vi "Find Tests from Path.vi"(8 "error in (no error)":errorcluster, 10 "Project or Class Path":path, 11 "Test Case Finder In":refnum<class "Indexing Test Finder.lvclass">) -> (0 "error out":errorcluster, 3 "Test Case Finder Out":refnum<class "Indexing Test Finder.lvclass">)   [LabVIEW 2020, in "Indexing Test Finder.lvclass"]
uses:
  Indexing Test Finder.lvclass
  Test Finder/Test Finder.lvclass
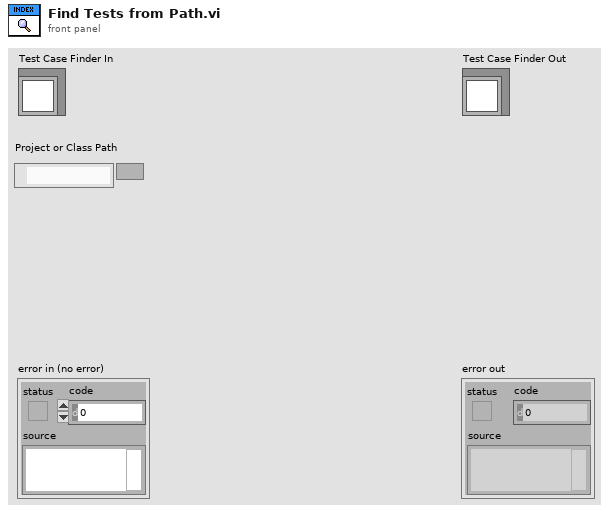
[diagram p1: front panel]
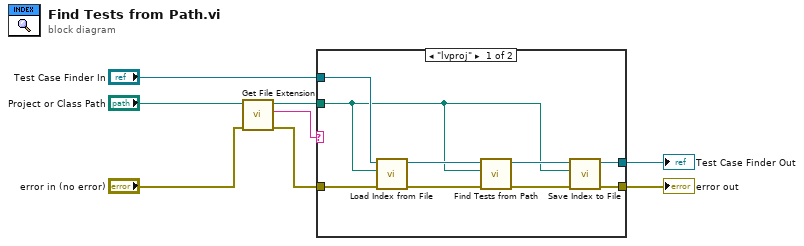
[diagram p0: block diagram]
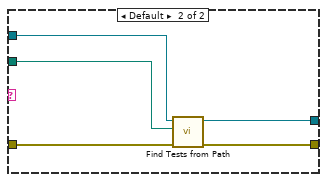
[diagram p2: hidden frame]
diagram:
  n1 = call <vilib>:"Get File Extension.vi"("error in (no error)"="error in (no error)", "file"="Project or Class Path") -> ("error out"=w4:errorcluster, "lowercase file extension"=w1:string, "dup file"=w2:path)  [unwired: 5 in, 2 out]
  n2 = case shown="\"lvproj\"" w1 {
    tunnel: "Test Case Finder In" -> [w17 w22]
    tunnel: [w13 w21] -> w6
    tunnel: [w11 w20] -> w5
    tunnel: w4 -> [w10 w19]
    tunnel: w2 -> [w9 w18]
    frame "lvproj" {
      n3 = call "Load Index from File.vi"("error in (no error)"=w10, "Project or Class Path"=w9, "Bufferend Test Finder in"=w17) -> ("error out"=w15:errorcluster, "Bufferend Test Finder out"=w16:refnum<class "Indexing Test Finder.lvclass">)  [unwired: 7 in]
      n4 = call-parent "Find Tests from Path.vi"("error in (no error)"=w15, "Project or Class Path"=w9, "Test Case Finder In"=w16) -> ("error out"=w12:errorcluster, "Test Case Finder Out"=w14:refnum<class "Indexing Test Finder.lvclass">)  [unwired: 7 in]
      n5 = call "Save Index to File.vi"("error in (no error)"=w12, "Project or Class Path"=w9, "Bufferend Test Finder in"=w14) -> ("error out"=w11:errorcluster, "Bufferend Test Finder out"=w13:refnum<class "Indexing Test Finder.lvclass">)  [unwired: 7 in]
    }
    frame Default {
      n6 = call-parent "Find Tests from Path.vi"("error in (no error)"=w19, "Project or Class Path"=w18, "Test Case Finder In"=w22) -> ("error out"=w20:errorcluster, "Test Case Finder Out"=w21:refnum<class "Indexing Test Finder.lvclass">)  [unwired: 7 in]
    }
  }
  "error out" <- w5
  "Test Case Finder Out" <- w6
